vi "Sub-FirstMeasurement.vi"(9 "time target (s)":dbl) -> (4 "誤差百分比":dbl, 5 "感測器壽命(天)":dbl, 11 "pH感測器異常":bool)   [LabVIEW 2017]
uses:
  <vilib>/myRIO/Instrument Drivers/Onboard IO/AI/typedefs/AI Reference.ctl
  <vilib>/myRIO/Common/Instrument Driver Framework/Utilities/typedefs/myRIO Generic Hardware Reference.ctl
  <vilib>/myRIO/Common/Instrument Driver Framework/Utilities/typedefs/Hardware Version Enum.ctl
  <vilib>/myRIO/Common/Instrument Driver Framework/Utilities/typedefs/myRIO v1.0 Reference.ctl
  <vilib>/myRIO/Common/Instrument Driver Framework/Utilities/typedefs/Generic FPGA Reference.ctl
  <vilib>/myRIO/Common/Instrument Driver Framework/myRIO v1.0/AI/typedefs/AI Channels List.ctl
  <vilib>/myRIO/Common/Instrument Driver Framework/myRIO v1.0/AI/typedefs/AI Channels Enum.ctl
  <vilib>/myRIO/Common/Instrument Driver Framework/Utilities/typedefs/Analog Scaling Constants List.ctl
  <vilib>/myRIO/Common/Instrument Driver Framework/Utilities/typedefs/Analog Scaling Constants.ctl
  <vilib>/userdefined/High Color/nirio_resource_hc.ctl
  <vilib>/myRIO/Common/Instrument Driver Framework/myRIO v1.0/AI/vis/myRIO v1.1 Open AI.vi
  <vilib>/myRIO/Common/Instrument Driver Framework/Utilities/vis/Validate Channels.vi
  <vilib>/myRIO/Common/Instrument Driver Framework/myRIO v1.0/AI/vis/myRIO v1.0 Reserve AI.vi
  <vilib>/myRIO/Common/Instrument Driver Framework/myRIO v1.0/AI/vis/myRIO v1.0 Close AI.vi
  <vilib>/myRIO/Common/Instrument Driver Framework/myRIO v1.0/AI/vis/myRIO v1.0 Build MUX Configuration AI.vi
  <vilib>/myRIO/Common/Instrument Driver Framework/myRIO v1.0/Resource Manager/vis/myRIO v1.0 Reserve Channel List.vi
  <vilib>/myRIO/Common/Instrument Driver Framework/myRIO v1.0/AI/vis/myRIO v1.0 Unreserve AI.vi
  <vilib>/myRIO/Common/Instrument Driver Framework/myRIO v1.0/Resource Manager/vis/myRIO v1.0 Reserve Channel.vi
  <vilib>/myRIO/Common/Instrument Driver Framework/myRIO v1.0/Resource Manager/vis/myRIO v1.0 Unreserve Channel.vi
  <vilib>/myRIO/Common/Instrument Driver Framework/myRIO v1.0/Resource Manager/vis/myRIO v1.0 Unreserve Channel List.vi
  <vilib>/myRIO/Common/Instrument Driver Framework/myRIO v1.0/Resource Manager/vis/myRIO v1.0 Build Mutex Name.vi
  <vilib>/Utility/VariantDataType/GetNumericInfo.vi
  <vilib>/Utility/error.llb/Error Cluster From Error Code.vi
  <vilib>/myRIO/Common/Instrument Driver Framework/myRIO v1.0/myRIO v1.1 Open.vi
  <vilib>/myRIO/Common/Instrument Driver Framework/myRIO v1.0/AI/vis/myRIO v1.0 Get Scaling Constants AI.vi
  <vilib>/myRIO/Common/Instrument Driver Framework/Utilities/vis/IO Manager.vi
  <vilib>/myRIO/Common/Instrument Driver Framework/Utilities/vis/Configuration Manager.vi
  <vilib>/myRIO/Common/Instrument Driver Framework/myRIO v1.0/myRIO v1.0 Close.vi
  <vilib>/myRIO/Common/Instrument Driver Framework/myRIO v1.0/AI/vis/myRIO v1.0 Read AI.vi
  <vilib>/myRIO/Instrument Drivers/Onboard IO/AI/vis/myRIO AI Open.xnode
  <vilib>/myRIO/Instrument Drivers/Onboard IO/AI/AI.lvlib
panel:
  out "Elapsed Time":dbl format="%.1g"
  out "pH_Voltage(mv)":dbl
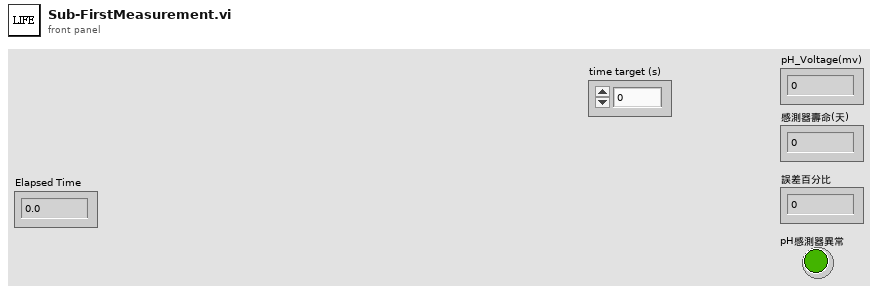
[diagram p1: front panel]
types:
  T1 = typedef "AI.lvlib/AI Reference.ctl" = cluster{"myRIO Reference":T2, "AI Channels List":T6, "AI Scaling Constants List":T8}
  T2 = typedef "myRIO Generic Hardware Reference.ctl" = cluster{"myRIO Model":T3, "myRIO Hardware Reference":T4}
  T3 = typedef "Hardware Version Enum.ctl" = enum16{"Unknown", "myRIO-1900", "myRIO-1950", "roboRIO", "NI ELVIS RIO CM"}
  T4 = typedef "myRIO v1.0 Reference.ctl" = cluster{"Generic FPGA Reference":T5, "Allow multiple opens":bool}
  T5 = typedef "Generic FPGA Reference.ctl" = refnum<k20>
  T6 = typedef "AI Channels List.ctl" = T7[]
  T7 = typedef "AI Channels Enum.ctl" = enum16{"Not Connected", "AudioIn/Left", "AudioIn/Right", "C/AI0", "C/AI1", "A/AI0", "A/AI1", "A/AI2", "A/AI3", "B/AI0", "B/AI1", "B/AI2", "B/AI3", "AI/AI0", "AI/AI1", "AI/AI2", "AI/AI3"}
  T8 = typedef "Analog Scaling Constants List.ctl" = T9[]
  T9 = typedef "Analog Scaling Constants.ctl" = cluster{"LSB Weight (Volts)":dbl, "Offset (Volts)":dbl, "Signed?":bool}
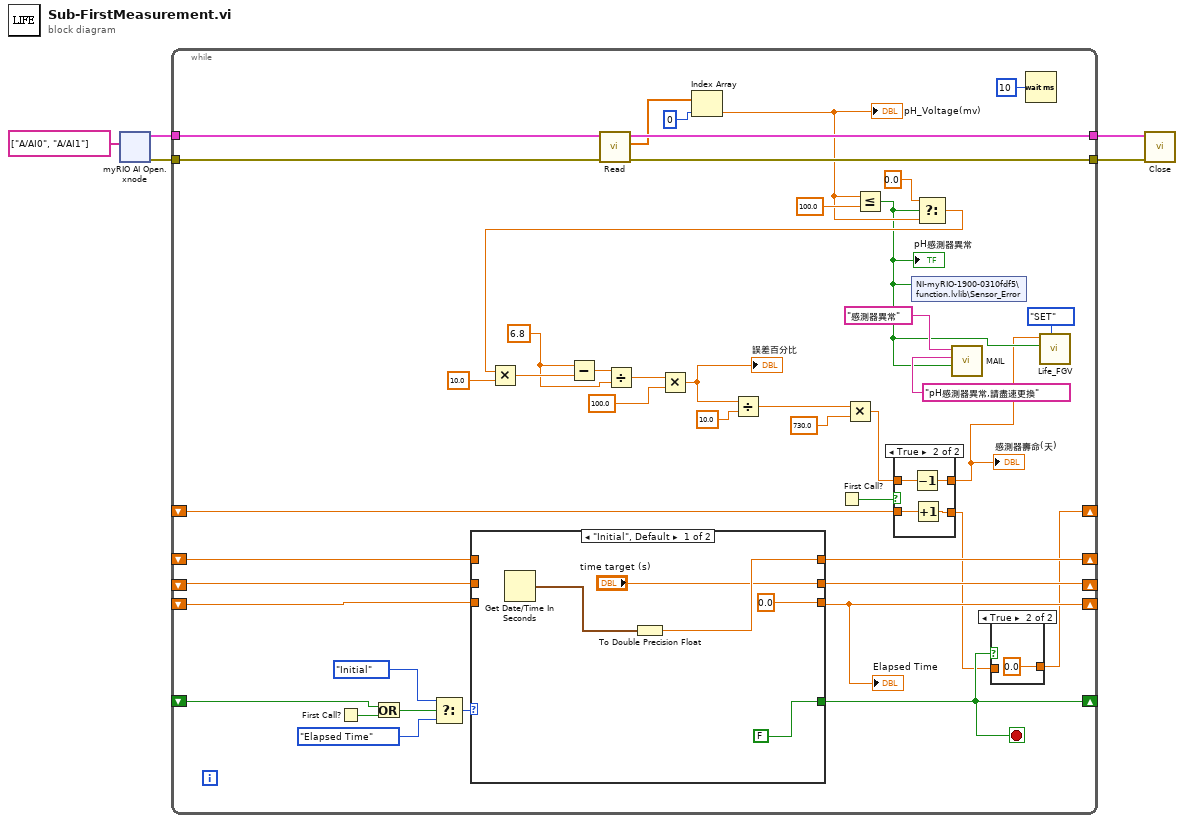
[diagram p0: block diagram]
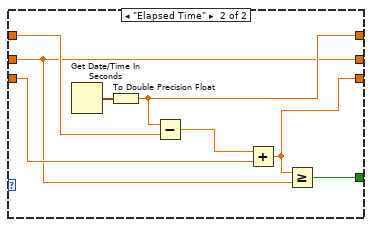
[diagram p4: hidden frame]
diagram:
  n1 = xnode "myRIO AI Open.xnode"("Channel Names"=tag[] ["A/AI0", "A/AI1"]) -> ("error out"=w4:errorcluster, "AI Ref Out"=w5:T1)  [unwired: 2 in]
  n2 = while {
    tunnel: w5 -> [w42]
    tunnel: w4 -> [w41]
    tunnel: [w40] -> w3
    tunnel: [w39] -> w2
    shift-right: [w29] -> _
    shift-left: _ -> [w32]
    shift-right: [w28] -> _
    shift-left: _ -> [w31]
    shift-right: [w27] -> _
    shift-left: _ -> [w30]
    shift-right: [w8] -> _
    shift-left: _ -> [w26]
    shift-right: [w7] -> _
    shift-left: _ -> [w9]
    stop <- w8 stop-if-true
    w14 = 6.8
    n3 = First Call?() -> (First Call?: T/F=w33:bool)
    n4 = Or(x=w26, y=w33) -> (x .or. y?=w34:bool)
    n5 = Select(t=enum16{"Initial", "Elapsed Time"}."Initial", s=w34, f=enum16{"Initial", "Elapsed Time"}."Elapsed Time") -> (s? t:f=w35:enum16{"Initial", "Elapsed Time"})
    n6 = case shown="\"Initial\", Default" w35 {
      tunnel: ["time target (s)" w65] -> w28
      tunnel: w31 -> [_ w65]
      tunnel: [w60 w68] -> w29
      tunnel: w32 -> [_ w69]
      tunnel: [0.0 w64] -> w27
      tunnel: w30 -> [_ w67]
      tunnel: [FALSE w66] -> w8
      frame "Initial", Default {
        n7 = Get Date/Time In Seconds() -> (seconds since 1Jan1904=w61:timestamp)
        n8 = To Double Precision Float(number=w61) -> (double precision float=w60:dbl)
      }
      frame "Elapsed Time" {
        n9 = Get Date/Time In Seconds() -> (seconds since 1Jan1904=w70:timestamp)
        n10 = To Double Precision Float(number=w70) -> (double precision float=w68:dbl)
        n11 = Subtract(x=w68, y=w69) -> (x-y=w63:dbl)
        n12 = Add(x=w63, y=w67) -> (x+y=w64:dbl)
        n13 = Greater Or Equal?(x=w64, y=w65) -> (x >= y?=w66:bool)
      }
    }
    "Elapsed Time" <- w27
    n14 = call <vilib>:"Read.vi"("error in (no error)"=w41, "AI Ref In"=w42) -> ("error out"=w39:errorcluster, "Values"=w38:dbl[], "AI Ref Out"=w40:T1)  [unwired: 7 in]
    n15 = Index Array(array=w38, index=0) -> (element=w21:dbl)
    "pH_Voltage(mv)" <- w21
    n16 = First Call?() -> (First Call?: T/F=w12:bool)
    n17 = Less Or Equal?(x=w21, y=100.0) -> (x <= y?=w16:bool)
    "pH感測器異常" <- w16
    n18 = shared-variable "NI-myRIO-1900-0310fdf5\\function.lvlib\\Sensor_Error"(w16) -> ()  [unwired: 1 in, 1 out]
    n19 = Select(t=0.0, s=w16, f=w21) -> (s? t:f=w23:dbl)
    n20 = Multiply(x=w23, y=10.0) -> (x*y=w15:dbl)
    n21 = Subtract(x=w14, y=w15) -> (x-y=w48:dbl)
    n22 = Divide(x=w48, y=w14) -> (x/y=w47:dbl)
    n23 = Multiply(x=w47, y=100.0) -> (x*y=w45:dbl)
    "誤差百分比" <- w45
    n24 = Divide(x=w45, y=10.0) -> (x/y=w13:dbl)
    n25 = Multiply(x=w13, y=730.0) -> (x*y=w11:dbl)
    n26 = case shown="True" w12 {
      tunnel: w11 -> [w53 w57]
      tunnel: [w53 w56] -> w10
      tunnel: w9 -> [w52 w55]
      tunnel: [w52 w54] -> w6
      frame False {
      }
      frame True {
        n27 = Decrement(x=w57) -> (x-1=w56:dbl)
        n28 = Increment(x=w55) -> (x+1=w54:dbl)
      }
    }
    "感測器壽命(天)" <- w10
    n29 = call "MAIL.vi"("寄送"=w16, "內容"="pH感測器異常,請盡速更換", "標題"="感測器異常") -> ()  [unwired: 9 in]
    n30 = case shown="True" w8 {
      tunnel: [w50 0.0 ("y")] -> w7
      tunnel: w6 -> [w50 _]
      frame False {
      }
      frame True {
      }
    }
    n31 = Wait (ms)(milliseconds to wait=u32 10) -> ()  [unwired: 1 out]
    n32 = call "Life_FGV.vi"("Command"=enum16{"SET", "GET"}."SET", "Error_IN"=w16, "Life_Value_IN"=w10) -> ()  [unwired: 6 in, 3 out]
  }
  n33 = call <vilib>:"Close.vi"("error in (no error)"=w2, "AI Ref In"=w3) -> ()  [unwired: 9 in, 1 out]
